vi "ConvertSize.vi"(11 "read buffer":string) -> (2 "# bytes":u32, 3 "size()":u32[](array[numeric]))   [LabVIEW 2022 SP3]
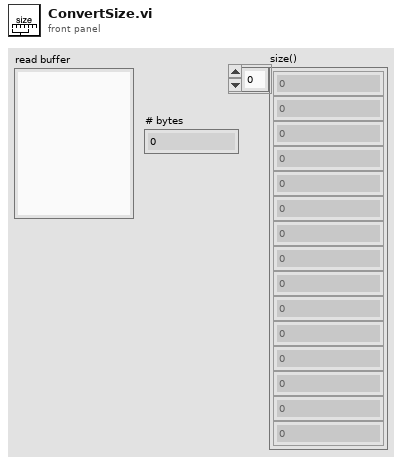
[diagram p1: front panel]
types:
  T1 = enum16{"big-endian, network order", "native, host order", "little-endian"}
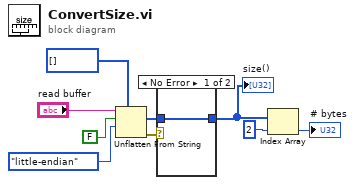
[diagram p0: block diagram]
diagram:
  n1 = Unflatten From String(type=u32[] [], binary string="read buffer", data includes array or string size? (T)=FALSE, byte order (0:big-endian, network order)=T1."little-endian") -> (value=w2:u32[], error out=w4:errorcluster)  [unwired: 1 in, 1 out]
  n2 = case shown="No Error" w4 {
    tunnel: [w10 _] -> w3
    tunnel: w2 -> [w10 _]
    frame No Error {
    }
    frame Error {
    }
  }
  "size()" <- w3
  n3 = Index Array(array=w3, index=2) -> (element=→"# bytes":u32)
